vi "PcData.vi"() -> ()   [LabVIEW 2016]
uses:
  <vilib>/Utility/file.llb/Write Delimited Spreadsheet (I64).vi
  <vilib>/ErrorRing/Error Ring.xnode
  <resource>/objmgr/ni.dex.rc
panel:
  in  "Channels":i32=16
  out "16通道波形":u16[][](graph)
  out "错误显示":errorcluster
  out "网络流缓存区数据量":i32
  in  "file path (dialog if empty)":path=path "E:/测试数据/新芯片"
  in  "存盘":bool
  out "max(x,y)":i32
  in  "stop":bool
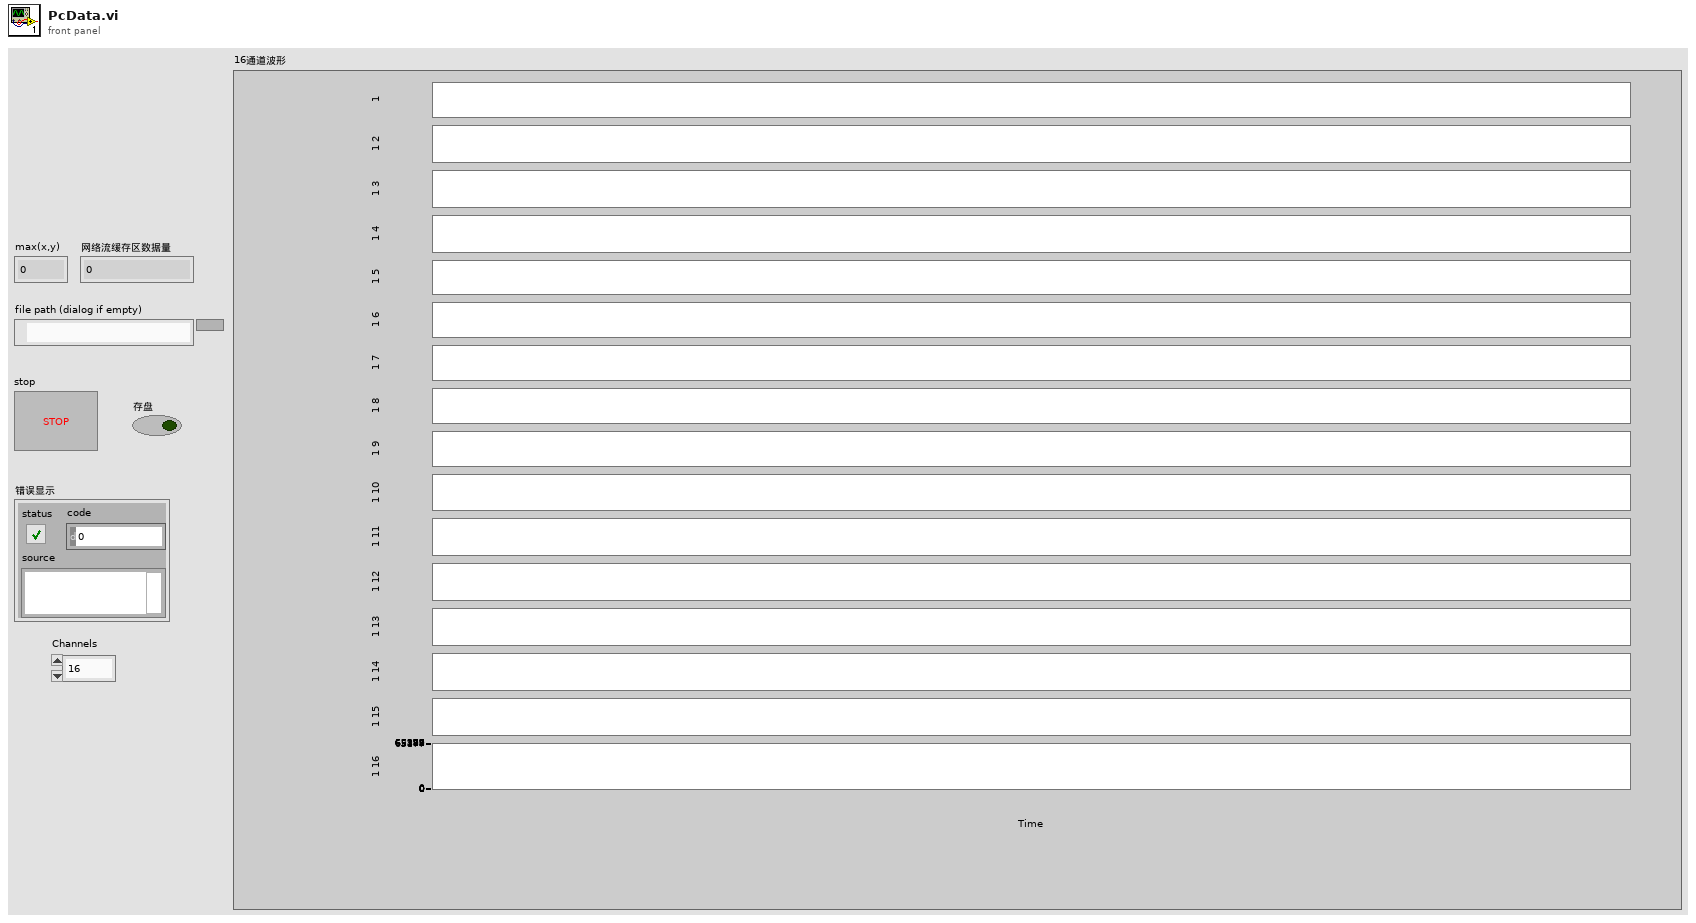
[diagram p1: front panel]
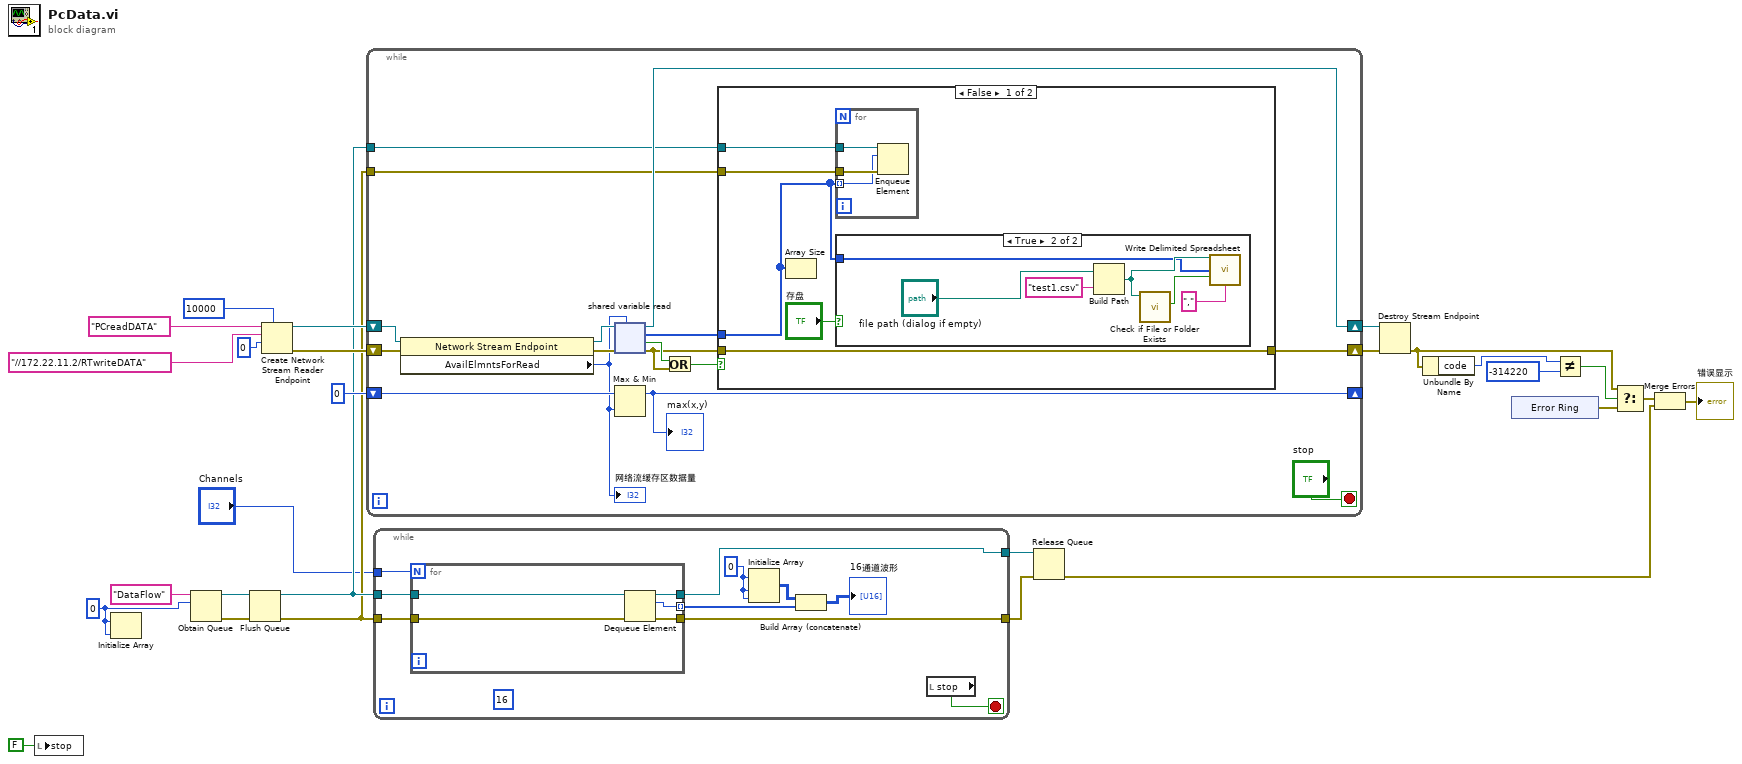
[diagram p0: block diagram]
diagram:
  w12 = u16 0
  n1 = local write "stop"(FALSE ("stop")) -> ()
  n2 = Initialize Array(w12, w12) -> ()  [unwired: 1 out]
  n3 = Obtain Queue(name (unnamed)="DataFlow", element data type=w12) -> (queue out=w11:refnum<queue>, error out=w9:errorcluster)  [unwired: 3 in, 1 out]
  n4 = Flush Queue(queue=w11, error in (no error)=w9) -> (queue out=w10:refnum<queue>, error out=w8:errorcluster)  [unwired: 1 out]
  n5 = Create Network Stream Reader Endpoint(7:10000 ("reader buffer size"), 9:u16 0 ("element"), 10:"//172.22.11.2/RTwriteDATA" ("writer url"), 11:"PCreadDATA" ("reader name")) -> (0:w25:errorcluster, 3:w24:refnum<k21>)  [unwired: 3 in]
  n6 = while {
    shift-right: [w35] -> w22
    shift-left: w25 -> [w42]
    shift-right: [w36] -> w23
    shift-left: w24 -> [w43]
    tunnel: w10 -> [w34]
    tunnel: w8 -> [w33]
    shift-right: [w29] -> _
    shift-left: 0 -> [w31]
    stop <- "stop" stop-if-true
    n7 = property class="Network Stream Endpoint"(reference=w43, error in=w42) -> (reference out=w41:refnum<k21>, error out=w40:errorcluster, "AvailElmntsForRead"=w30:i32)
    "网络流缓存区数据量" <- w30
    n8 = shared-variable-read(w41, w40, w30) -> (w36:refnum<k21>, w37:errorcluster, w38:bool, w32:u16[])  [unwired: 1 in]
    n9 = Max & Min(x=w31, y=w30) -> (max(x,y)=w29:i32)  [unwired: 1 out]
    "max(x,y)" <- w29
    n10 = Or(x=w38, y=w37) -> (x .or. y?=w39:bool)
    n11 = case shown="False" w39 {
      tunnel: w37 -> [w48 w58]
      tunnel: [w48 w58] -> w35
      tunnel: w32 -> [w44 _]
      tunnel: w34 -> [w47 _]
      tunnel: w33 -> [w46 _]
      frame False {
        n12 = Array Size(array=w44) -> ()  [unwired: 1 out]
        n13 = for {
          tunnel: w47 -> [w51]
          tunnel: w46 -> [w50]
          tunnel: w44 -> [w49] mode=indexing
          n14 = Enqueue Element(queue=w51, element=w49, error in (no error)=w50) -> ()  [unwired: 1 in, 3 out]
        }
        n15 = case shown="True" "存盘" {
          tunnel: w44 -> [_ w53]
          frame False {
          }
          frame True {
            n16 = Build Path(base path="file path (dialog if empty)", name or relative path="test1.csv") -> (appended path=w56:path)
            n17 = call <vilib>:"Check if File or Folder Exists.vi"("path"=w56) -> ("file or folder exists?"=w55:bool)  [unwired: 8 in, 2 out]
            n18 = call-poly <vilib>:"Write Delimited Spreadsheet.vi"("file path (dialog if empty)"=w56, "1D data"=w53, "append to file? (new file:F)"=w55, "delimiter (\\t)"="," ("delimiter (\\t)")) -> ()  [unwired: 10 in, 2 out]
          }
        }
      }
      frame True {
      }
    }
  }
  n19 = while {
    tunnel: w10 -> [w68]
    tunnel: w8 -> [w63]
    tunnel: [w62] -> w7
    tunnel: [w61] -> w6
    tunnel: "Channels" -> [w59]
    stop <- w60 stop-if-true
    w67 = u16 0
    (unwired) 16
    n20 = for {
      N: w59 -> [_]
      tunnel: w68 -> [w73]
      tunnel: [w72] -> w65 mode=indexing
      tunnel: w63 -> [w71]
      tunnel: [w70] -> w62
      tunnel: [w69] -> w61
      n21 = Dequeue Element(queue=w73, error in (no error)=w71) -> (queue out=w70:refnum<queue>, element=w72:u16, error out=w69:errorcluster)  [unwired: 1 in, 1 out]
    }
    n22 = Initialize Array(w67, w67, w67) -> (w66:u16[][])
    n23 = Build Array (concatenate)(w66, w65) -> (→"16通道波形":u16[][])
    n24 = local read "stop"() -> (w60:bool)
  }
  n25 = Release Queue(queue=w7, error in (no error)=w6) -> (error out=w4:errorcluster)  [unwired: 1 in, 2 out]
  n26 = Destroy Stream Endpoint(8:w22, 11:w23) -> (0:w16:errorcluster)
  n27 = Unbundle By Name(w16) -> ("code"=w20:i32)
  n28 = xnode "Error Ring"() -> ("error out"=w17:errorcluster)
  n29 = Not Equal?(x=w20, y=-314220) -> (x != y?=w18:bool)
  n30 = Select(t=w16, s=w18, f=w17) -> (s? t:f=w5:errorcluster)
  n31 = Merge Errors(w5, w4) -> (→"错误显示":errorcluster)
